vi "Get List of Names.vi"(8 "error in (no error)":errorcluster, 11 "FPGA Interface in":refnum<class "FPGA Interface.lvclass">) -> (0 "error out":errorcluster, 1 "List of IPs":string[](array[string]), 2 "List of Names":string[](array[string]), 3 "FPGA Interface out":refnum<class "FPGA Interface.lvclass">)   [LabVIEW 2026, in "TALOS.lvlib" / "Interfaces.lvlib" / "FPGA Interface.lvclass"]
uses:
  FPGA Interface.lvclass
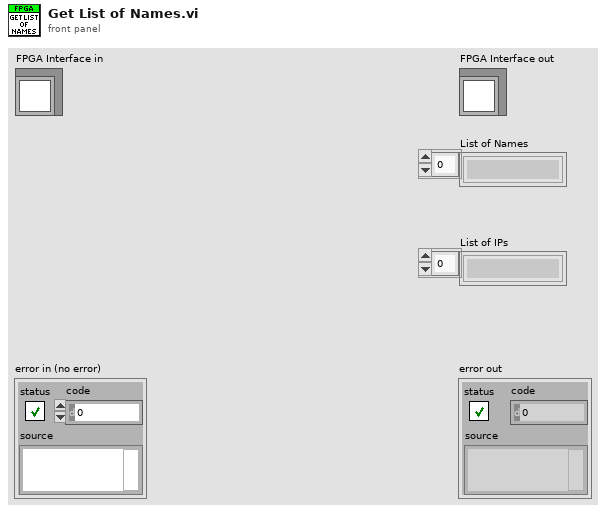
[diagram p1: front panel]
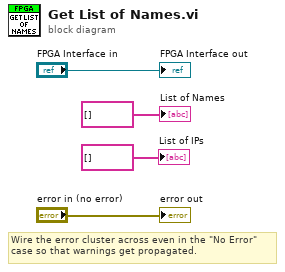
[diagram p0: block diagram]
diagram:
  # "Wire the error cluster across even in the \"No Error\"\ncase so that warnings get propagated."
  "error out" <- "error in (no error)"
  "FPGA Interface out" <- "FPGA Interface in"
  "List of Names" <- string[] [] ("List of Names")
  "List of IPs" <- string[] [] ("List of IPs")
